vi "TCP-Send Command Receive String.vi"(0 "PXI Address":string, 5 "Port":i32, 7 "Command":string, 9 "timeout (ms)":i32=5000, 11 "error in (no error)":errorcluster) -> (4 "data":string, 10 "result":i32, 15 "error out":errorcluster)   [LabVIEW 2020]
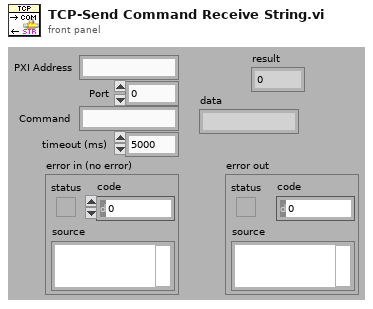
[diagram p1: front panel]
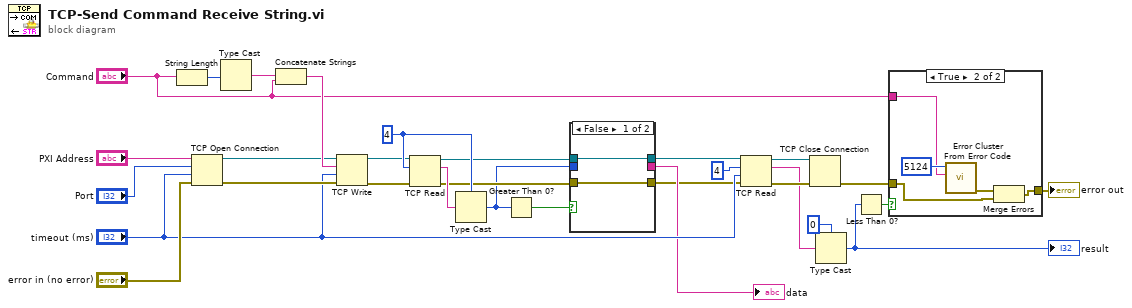
[diagram p0: block diagram]
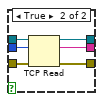
[diagram p2: hidden frame]
diagram:
  w10 = 4
  n1 = String Length(string="Command") -> (length=w26:i32)
  n2 = TCP Open Connection(address="PXI Address", remote port or service name="Port", timeout ms (60000)="timeout (ms)", error in (no error)="error in (no error)") -> (connection ID=w23:refnum<k5>, error out=w24:errorcluster)  [unwired: 1 in]
  n3 = Type Cast(x=w26) -> (*(type *) &x=w25:string)  [unwired: 1 in]
  n4 = Concatenate Strings(w25, "Command") -> (w27:string)
  n5 = TCP Write(connection ID=w23, data in=w27, error in (no error)=w24, 9:"timeout (ms)") -> (connection ID out=w9:refnum<k5>, error out=w8:errorcluster)  [unwired: 1 out]
  n6 = TCP Read(connection ID=w9, bytes to read=w10, error in (no error)=w8) -> (connection ID out=w6:refnum<k5>, data out=w11:string, error out=w7:errorcluster)  [unwired: 2 in]
  n7 = Type Cast(type=w10, x=w11) -> (*(type *) &x=w3:i32)
  n8 = Greater Than 0?(x=w3) -> (x > 0?=w2:bool)
  n9 = case shown="False" w2 {
    tunnel: [_ w38] -> w4
    tunnel: [w32 w37] -> w1
    tunnel: w6 -> [w31 w36]
    tunnel: w7 -> [w32 w35]
    tunnel: w3 -> [_ w34]
    tunnel: [w31 w33] -> w5
    frame False {
    }
    frame True {
      n10 = TCP Read(connection ID=w36, bytes to read=w34, error in (no error)=w35) -> (connection ID out=w33:refnum<k5>, data out=w38:string, error out=w37:errorcluster)  [unwired: 2 in]
    }
  }
  "data" <- w4
  n11 = TCP Read(connection ID=w5, bytes to read=4, error in (no error)=w1, 9:"timeout (ms)") -> (connection ID out=w19:refnum<k5>, data out=w18:string, error out=w20:errorcluster)  [unwired: 1 in]
  n12 = TCP Close Connection(connection ID=w19, error in (no error)=w20) -> (error out=w13:errorcluster)  [unwired: 1 in, 1 out]
  n13 = Type Cast(type=0, x=w18) -> (*(type *) &x=w16:i32)
  "result" <- w16
  n14 = Less Than 0?(x=w16) -> (x < 0?=w15:bool)
  n15 = case shown="True" w15 {
    tunnel: [w39 w41] -> w14
    tunnel: w13 -> [w39 w40]
    tunnel: "Command" -> [_ w42]
    frame False {
    }
    frame True {
      n16 = call <vilib>:"Error Cluster From Error Code.vi"("error message (\"\")"=w42, "error code (0)"=5124) -> ("error out"=w44:errorcluster)  [unwired: 7 in]
      n17 = Merge Errors(w44, w40) -> (w41:errorcluster)
    }
  }
  "error out" <- w14
